vi "Get Input.vi"(11 "Reply Msg DataSocket Simple in":refnum<class "Reply Msg DataSocket Simple.lvclass">) -> (2 "Input":variant, 3 "Reply Msg DataSocket Simple out":refnum<class "Reply Msg DataSocket Simple.lvclass">)   [LabVIEW 2023, in "Reply Msg DataSocket Simple.lvclass"]
uses:
  Reply Msg DataSocket Simple.lvclass
  Reply Msg DataSocket Simple.lvclass/Reply Msg DataSocket Simple.ctl
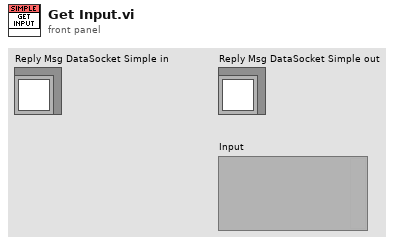
[diagram p1: front panel]
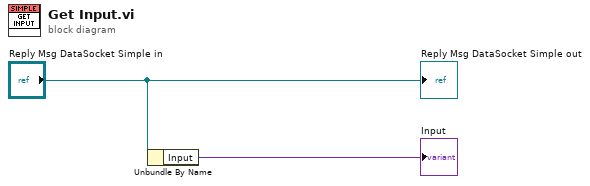
[diagram p0: block diagram]
diagram:
  n1 = Unbundle By Name("Reply Msg DataSocket Simple in") -> ("Input"=→"Input":variant)
  "Reply Msg DataSocket Simple out" <- "Reply Msg DataSocket Simple in"
